vi "LIN State to String.vi"(11 "LIN comm in":T1 {"communication state" items=["Idle", "Active", "Inactive"]; "fault code" format="%08x"; "last error" items=["None", "Unknown ID", "Form", "Framing", "Readback", "Timeout", "Checksum"]}) -> (3 "string out":string)   [LabVIEW 2025, in "CAN-LIN Raw Bus Capture.lvclass"]
uses:
  <vilib>/xnet/xnet.llb/XNET LIN Comm.ctl
  <vilib>/xnet/xnet.llb/XNET LIN Comm State.ctl
  <vilib>/xnet/xnet.llb/XNET LIN Last Err.ctl
  CAN-LIN Raw Bus Capture.lvclass
  CAN-LIN Raw Bus Capture.lvclass/CAN-LIN Raw Bus Capture.ctl
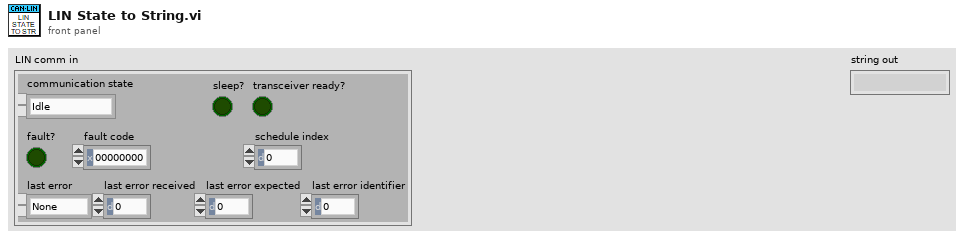
[diagram p1: front panel]
types:
  T1 = typedef "XNET LIN Comm.ctl" = cluster{"fault code":i32, "fault?":bool, "communication state":T2, "last error":T3, "last error received":u8, "last error expected":u8, "last error identifier":u8, "sleep?":bool, "transceiver ready?":bool, "schedule index":u8}
  T2 = typedef "XNET LIN Comm State.ctl" = u8
  T3 = typedef "XNET LIN Last Err.ctl" = u8
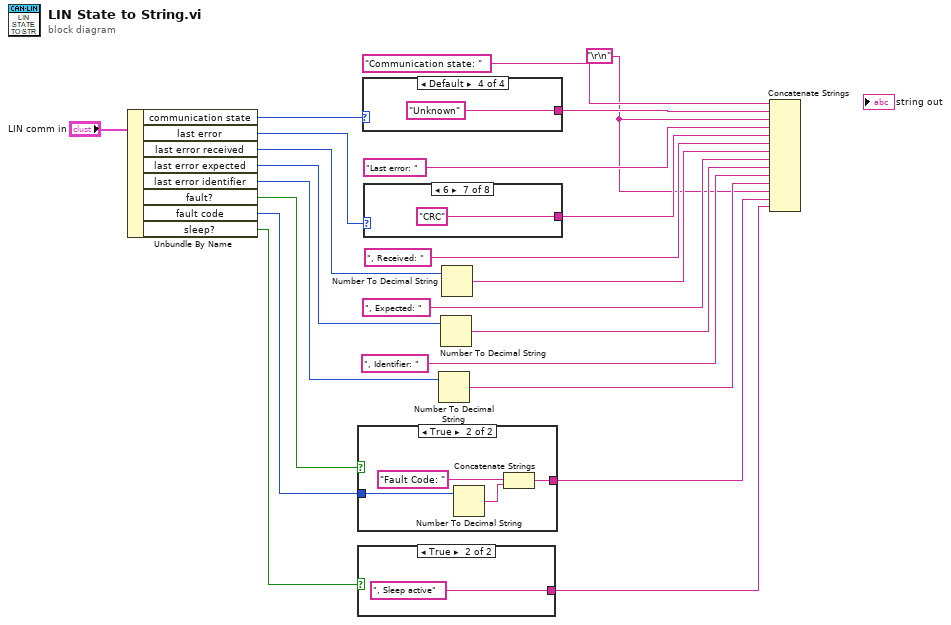
[diagram p0: block diagram]
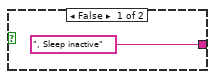
[diagram p2: hidden frame]
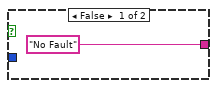
[diagram p3: hidden frame]
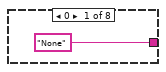
[diagram p4: hidden frame]
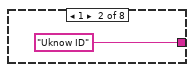
[diagram p5: hidden frame]
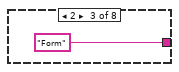
[diagram p6: hidden frame]
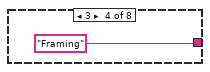
[diagram p7: hidden frame]
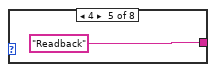
[diagram p8: hidden frame]
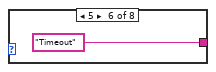
[diagram p9: hidden frame]
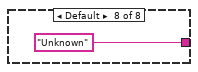
[diagram p10: hidden frame]
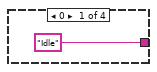
[diagram p11: hidden frame]
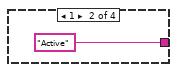
[diagram p12: hidden frame]
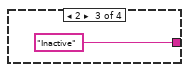
[diagram p13: hidden frame]
diagram:
  w6 = "\r\n"
  n1 = Unbundle By Name("LIN comm in") -> ("communication state"=w15:T2, "last error"=w14:T3, "last error received"=w13:u8, "last error expected"=w12:u8, "last error identifier"=w11:u8, "fault?"=w5:bool, "fault code"=w4:i32, "sleep?"=w3:bool)
  n2 = case shown="True" w5 {
    tunnel: w4 -> [_ w27]
    tunnel: ["No Fault" ("string") w24] -> w2
    frame False {
    }
    frame True {
      n3 = Number To Decimal String(number=w27) -> (decimal integer string=w25:string)  [unwired: 1 in]
      n4 = Concatenate Strings("Fault Code: " ("string"), w25) -> (w24:string)
    }
  }
  n5 = case shown="True" w3 {
    tunnel: [", Sleep inactive" ("string") ", Sleep active" ("string")] -> w1
    frame False {
    }
    frame True {
    }
  }
  n6 = case shown="Default" w15 {
    tunnel: ["Idle" ("string") "Active" ("string") "Inactive" ("string") "Unknown" ("string")] -> w21
    frame 0 {
    }
    frame 1 {
    }
    frame 2 {
    }
    frame Default {
    }
  }
  n7 = case shown="6" w14 {
    tunnel: ["None" ("string") "Uknow ID" ("string") "Form" ("string") "Framing" ("string") "Readback" ("string") "Timeout" ("string") "CRC" ("string") "Unknown" ("string")] -> w19
    frame 0 {
    }
    frame 1 {
    }
    frame 2 {
    }
    frame 3 {
    }
    frame 4 {
    }
    frame 5 {
    }
    frame 6 {
    }
    frame Default {
    }
  }
  n8 = Number To Decimal String(number=w11) -> (decimal integer string=w7:string)  [unwired: 1 in]
  n9 = Number To Decimal String(number=w12) -> (decimal integer string=w9:string)  [unwired: 1 in]
  n10 = Number To Decimal String(number=w13) -> (decimal integer string=w17:string)  [unwired: 1 in]
  n11 = Concatenate Strings("Communication state: " ("string"), w21, w6, "Last error: " ("string"), w19, ", Received: " ("string"), w17, ", Expected: " ("string"), w9, ", Identifier: " ("string"), w7, w6, w2, w1) -> ()  [unwired: 1 out]
